vi "picoquant_process_records.vi"(8 "error in (no error)":errorcluster, 10 "data":u32[](array[numeric]), 11 "hydraharp in":refnum<class "hydraharp.lvclass">) -> (0 "error out":errorcluster, 2 "data":T1, 3 "hydraharp out":refnum<class "hydraharp.lvclass">)   [LabVIEW 2015, in "hydraharp.lvclass"]
uses:
  hydraharp.lvclass
  Picoquant_generic/picoquant_data_tdef.ctl
  hydraharp.lvclass/hydraharp.ctl
  hydraharp_panel/hpanel_acq_modes.ctl
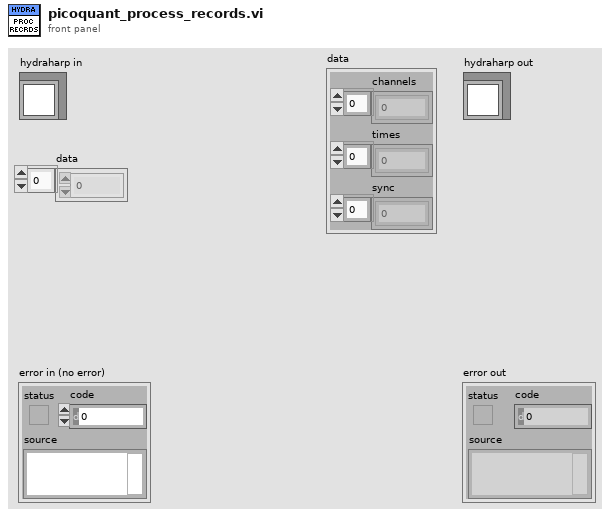
[diagram p1: front panel]
types:
  T1 = typedef "picoquant_data_tdef.ctl" = cluster{"channels":u8[], "times":u64[], "sync":u64[]}
  T2 = typedef "hpanel_acq_modes.ctl" = u16
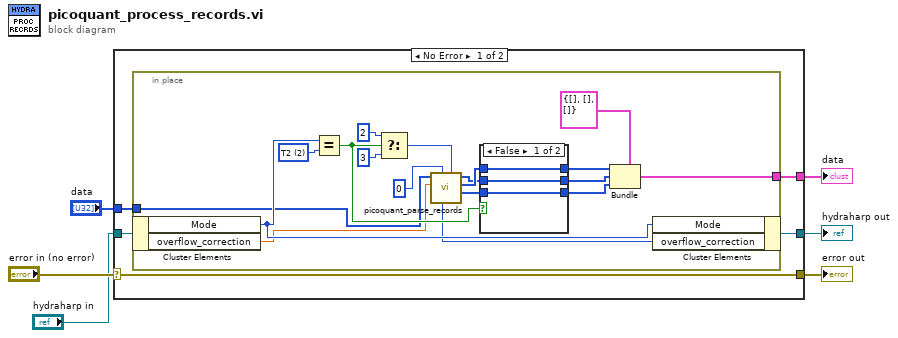
[diagram p0: block diagram]
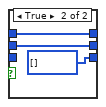
[diagram p2: hidden frame]
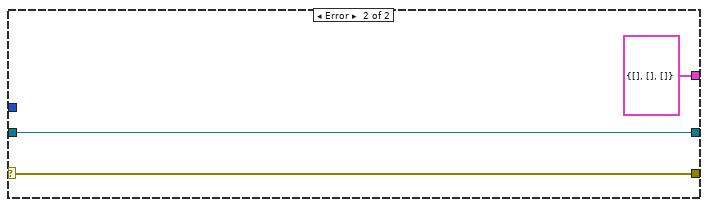
[diagram p3: hidden frame]
diagram:
  n1 = case shown="No Error" "error in (no error)" {
    selector: "error in (no error)" -> [w11 w38]
    tunnel: [w11 w38] -> w3
    tunnel: [w9 w37] -> w2
    tunnel: "hydraharp in" -> [w10 w37]
    tunnel: "data" -> [w8 _]
    tunnel: [w7 T1 {"channels"=[], "times"=[], "sync"=[]} ("output cluster")] -> w1
    frame No Error {
      n2 = in-place {
        in-place-border: w8 -> [w17]
        in-place-border: [w12] -> w7
        w29 = T2 2 items=["T2"=2, "T3"=3] ("Mode")
        n3 = in-place-cluster #1(w10) -> ("Mode"=w23:T2, "overflow_correction"=w20:dbl)
        n4 = Equal?(x=w23, y=w29) -> (x = y?=w22:bool)
        n5 = Select(t=u8 2 ("tmode"), s=w22, f=u8 3) -> (s? t:f=w18:u8)
        n6 = call "picoquant_parse_records.vi"("acq_mode"=w18, "Device"=u8 0 ("device"), "overflow"=w20, "fifo_buffer"=w17) -> ("sync"=w26:u64[], "channels"=w25:u8[], "times"=w24:u64[], "overflow"=w19:u64)  [unwired: 2 in, 2 out]
        n7 = case shown="False" w22 {
          tunnel: w26 -> [w30 _]
          tunnel: w25 -> [w31 w35]
          tunnel: w24 -> [w32 w34]
          tunnel: [w31 w35] -> w16
          tunnel: [w32 w34] -> w15
          tunnel: [w30 u64[] [] ("sync")] -> w14
          frame False {
          }
          frame True {
          }
        }
        n8 = Bundle(cluster=T1 {"channels"=[], "times"=[], "sync"=[]} ("output cluster"), "channels"=w16, "times"=w15, "sync"=w14) -> (w12:T1)
        n9 = in-place-cluster #1("Mode"=w23, "overflow_correction"=w19) -> (w9:refnum<class "hydraharp.lvclass">)
      }
    }
    frame Error {
    }
  }
  "error out" <- w3
  "hydraharp out" <- w2
  "data" <- w1
